vi "Get Pressure.vi"(8 "error in":errorcluster, 11 "PPT in":refnum<class "PPT.lvclass">) -> (0 "error out":errorcluster, 2 "Pressure":dbl, 3 "PPT out":refnum<class "PPT.lvclass">)   [LabVIEW 2014, in "PPT Library.lvlib" / "PPT.lvclass"]
doc: "Set the transceiver operating parameters. See PPT documentation to determine how the input parameter is applied."
uses:
  PPT.lvclass
  reusable/Session APIs/Serial/Serial Session.lvclass
  PPT.lvclass/PPT.ctl
  reusable/Session APIs/Serial/Public/Asynchronous Write.vi
  reusable/Session APIs/Serial/Public/Asynchronous Read.vi
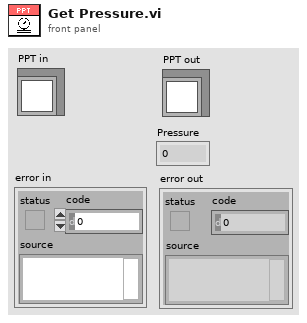
[diagram p1: front panel]
types:
  T1 = typedef "Session - Root.lvclass/Session Handle.ctl" = refnum<data-value>
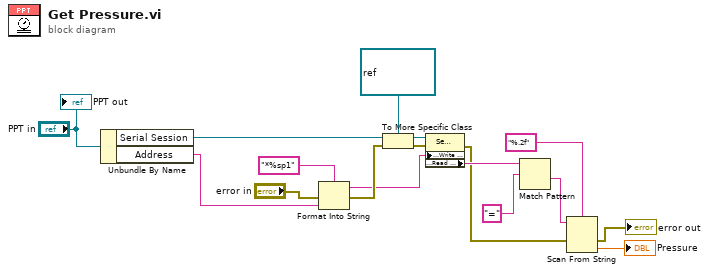
[diagram p0: block diagram]
diagram:
  n1 = Unbundle By Name("PPT in") -> ("Serial Session"=w4:T1, "Address"=w5:string)
  n2 = Format Into String(format string="*%sp1", error in="error in", w5) -> (resulting string=w6:string, error out=w7:errorcluster)  [unwired: 1 in]
  n3 = To More Specific Class(target class=refnum<data-value> refnum ("Serial Session"), reference=w4, error in=w7) -> (specific class reference=w10:refnum<data-value>, error out=w9:errorcluster)
  n4 = property class="Serial Session"(reference=w10, error in=w9, "Public:Write - Asynchronous"=w6) -> (error out=w2:errorcluster, "Public:Read - Asynchronous"=w14:string)  [unwired: 1 out]
  n5 = Match Pattern(string=w14, regular expression="=") -> (after substring=w12:string)  [unwired: 1 in, 3 out]
  n6 = Scan From String(format string="%.2f", input string=w12, error in=w2) -> (error out=→"error out":errorcluster, output 1=→"Pressure":dbl)  [unwired: 2 in, 2 out]
  "PPT out" <- "PPT in"
